vi "glownaMaszynaStanow.vi"(8 "Error in":errorcluster, 11 "Lista komór":T1[](array[typedef])) -> ()   [LabVIEW 2014]
uses:
  glownaMaszynaStanowVIs/wykonajRuchVIs/parametryKomorVIs/WyborKomory.ctl
  glownaMaszynaStanowVIs/Stan_glowny.ctl
  glownaMaszynaStanowVIs/AkcjaRuchu.ctl
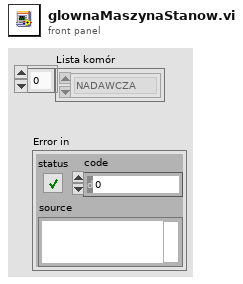
[diagram p1: front panel]
types:
  T1 = typedef "WyborKomory.ctl" = enum16{"NADAWCZA", "ODBIORCZA"}
  T2 = typedef "Stan_glowny.ctl" = enum16{"Oczekiwanie", "Init", "Działanie", "Koniec"}
  T3 = typedef "AkcjaRuchu.ctl" = enum16{"Init", "Reset ramienia", "Przygotuj listę", "Sprawdź", "Koniec"}
  T4 = typedef "WejsciaParametry.ctl" = cluster{"LEWO":bool, "PRAWO":bool, "GORA":bool, "DOL":bool, "Praca reczna":bool, "Stop":bool, "Start":bool, "Komora":bool, "Wyjscie":bool, "Rodzaj pomiarow":T5, "Czas pomiaru [s]":dbl, "Czas inicjalizacji ramion [s]":dbl, "Definicja punktów użytkownika":i32[][]}
  T5 = typedef "RodzajPomiarow.ctl" = enum16{"Izolacyjność Akustyczna ISO 10140", "Sekwencja testowa", "Definicja użytkownika"}
  T6 = typedef "LMH-LINX.lvlib/LINX Ref.ctl" = cluster{"IO":T7, "Interface":T8, "LINX Device Config":T9}
  T7 = typedef "LMH-LINX.lvlib/Platform.ctl" = enum16{"Remote", "Local"}
  T8 = typedef "LMH-LINX.lvlib/Interface.ctl" = enum16{"Serial", "TCP"}
  T9 = typedef "LMH-LINX.lvlib/Device.lvlib/LINX Device Config.ctl" = cluster{"Interface":T8, "COM Port":refnum<visa-resource-name>, "TCP Configuration":T10, "Device Family":u8, "Device ID":u8, "Device Name":string, "TCP Ref":refnum<k5>, "Channels":T11}
  T10 = typedef "LMH-LINX.lvlib/Device.lvlib/TCP Config.ctl" = cluster{"IP Address":string, "Port":u16}
  T11 = typedef "LMH-LINX.lvlib/Channels.ctl" = cluster{"DI":u8[], "DO":u8[], "AI":u8[], "AO":u8[], "PWM":u8[], "QE":u8[], "UART":u8[], "I2C 2":u8[], "SPI":u8[], "CAN":u8[], "Servo":u8[], "AI Ref (V)":dbl, "AI Resolution (Bits)":u8, "AO Ref (V)":dbl, "AO Resolution (Bits)":u8}
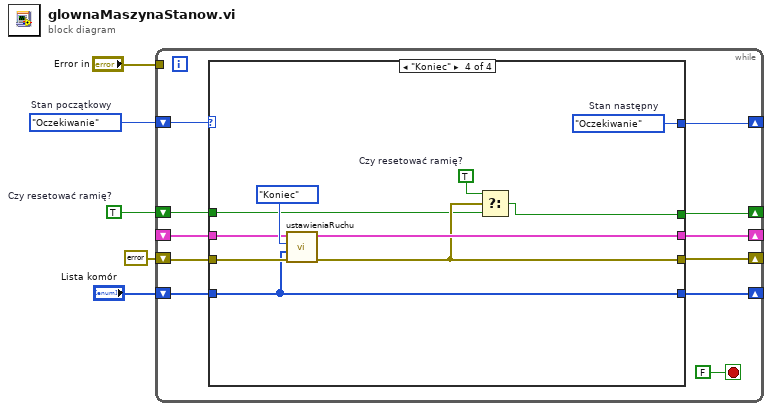
[diagram p0: block diagram]
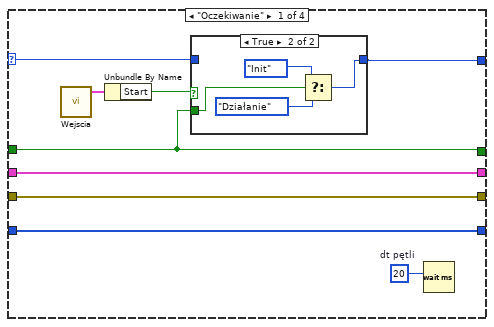
[diagram p2: hidden frame]
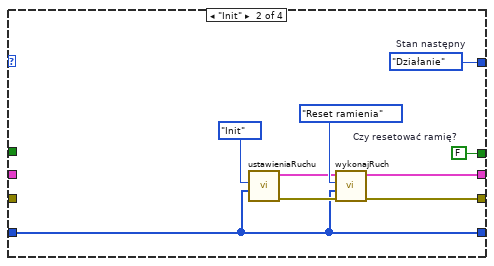
[diagram p4: hidden frame]
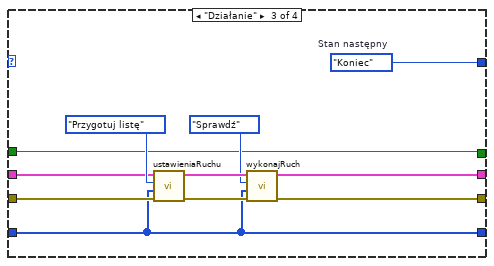
[diagram p5: hidden frame]
diagram:
  w4 = TRUE  # Czy resetować ramię?
  w5 = Stan_glowny."Oczekiwanie"  # Stan początkowy
  n1 = while {
    shift-right: [w12] -> _
    shift-left: w5 -> [w16]
    shift-right: [w10] -> _
    shift-left: w4 -> [w11]
    shift-right: [w13] -> _
    shift-left: _ -> [w15]
    shift-right: [w8] -> _
    shift-left: errorcluster {"status"=FALSE, "code"=0, "source"=""} ("error IO") -> [w14]
    shift-right: [w6] -> _
    shift-left: "Lista komór" -> [w9]
    tunnel: "Error in" -> [_]
    stop <- FALSE stop-if-true
    n2 = case shown="\"Koniec\"" w16 {
      selector: w16 -> [w20 _ _ _]
      tunnel: w15 -> [w24 _ w47 w58]
      tunnel: w14 -> [w25 _ w46 w57]
      tunnel: [w24 w39 w43 w56] -> w13
      tunnel: [w25 w38 w41 w54] -> w8
      tunnel: [w19 w37 w40 w60] -> w12
      tunnel: w11 -> [w18 _ w44 w53]
      tunnel: [w18 w32 w44 w51] -> w10
      tunnel: w9 -> [w22 w31 w42 w55]
      tunnel: [w22 w31 w42 w55] -> w6
      frame "Oczekiwanie" {
        w17 = u32 20  # dt pętli
        n3 = call "Wejscia.vi"() -> ("Wyjście"=w23:T4)  [unwired: 5 in]
        n4 = Unbundle By Name(w23) -> ("Start"=w21:bool)
        n5 = case shown="True" w21 {
          tunnel: w20 -> [w26 _]
          tunnel: [w26 w29] -> w19
          tunnel: w18 -> [_ w30]
          frame False {
          }
          frame True {
            n6 = Select(t=Stan_glowny."Init" ("Stan następny"), s=w30, f=Stan_glowny."Działanie") -> (s? t:f=w29:T2)
          }
        }
        n7 = Wait (ms)(milliseconds to wait=w17) -> ()  [unwired: 1 out]
      }
      frame "Init" {
        w32 = FALSE  # Czy resetować ramię?
        w37 = Stan_glowny."Działanie"  # Stan następny
        n8 = call "ustawieniaRuchu.vi"("Lista komór"=w31, "Rodzaj akcji"=AkcjaRuchu."Init" ("Akcja")) -> ("error out"=w33:errorcluster, "LINX Resource out"=w34:T6)  [unwired: 6 in]
        n9 = call "wykonajRuch.vi"("error in (no error)"=w33, "Lista komór"=w31, "Akcja"=AkcjaRuchu."Reset ramienia", "LINX Resource in"=w34) -> ("error out"=w38:errorcluster, "LINX Resource out"=w39:T6)  [unwired: 6 in]
      }
      frame "Działanie" {
        w40 = Stan_glowny."Koniec"  # Stan następny
        n10 = call "ustawieniaRuchu.vi"("error in"=w46, "Lista komór"=w42, "Rodzaj akcji"=AkcjaRuchu."Przygotuj listę" ("Akcja"), "LINX Resource in"=w47) -> ("error out"=w50:errorcluster, "LINX Resource out"=w49:T6)  [unwired: 4 in]
        n11 = call "wykonajRuch.vi"("error in (no error)"=w50, "Lista komór"=w42, "Akcja"=AkcjaRuchu."Sprawdź", "LINX Resource in"=w49) -> ("error out"=w41:errorcluster, "LINX Resource out"=w43:T6)  [unwired: 6 in]
      }
      frame "Koniec" {
        w52 = TRUE  # Czy resetować ramię?
        w60 = Stan_glowny."Oczekiwanie"  # Stan następny
        n12 = call "ustawieniaRuchu.vi"("error in"=w57, "Lista komór"=w55, "Rodzaj akcji"=AkcjaRuchu."Koniec", "LINX Resource in"=w58) -> ("error out"=w54:errorcluster, "LINX Resource out"=w56:T6)  [unwired: 4 in]
        n13 = Select(t=w52, s=w54, f=w53) -> (s? t:f=w51:bool)
      }
    }
  }
